vi "CmdData1.vi"() -> ()   [LabVIEW 2011]
panel:
  in  "Data1":dbl
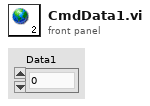
[diagram p1: front panel]
diagram:
